vi "I32toU8array.vi"(1 "I32":i32) -> (0 "U8":u8[](array[numeric]))   [LabVIEW 2021]
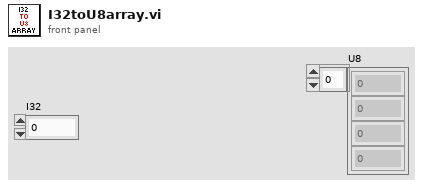
[diagram p1: front panel]
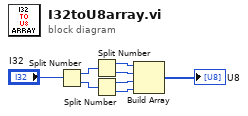
[diagram p0: block diagram]
diagram:
  n1 = Split Number(x="I32") -> (hi(x)=w7:u16, lo(x)=w8:u16)
  n2 = Split Number(x=w7) -> (hi(x)=w6:u8, lo(x)=w5:u8)
  n3 = Split Number(x=w8) -> (hi(x)=w4:u8, lo(x)=w3:u8)
  n4 = Build Array(w6, w5, w4, w3) -> (→"U8":u8[])
